vi "sub_get user input.vi"() -> (0 "Peltier Channels":i16[](array[numeric]), 1 "DAQ Sample Rate":dbl)   [LabVIEW 2021]
uses:
  globalvariables.vi
panel:
  in  "Peltier 2":i16(ring)=4 items=["N/A"=-1, "COM 1"=1, "COM 4"=4]
  in  "Peltier 1":i16(ring)=1 items=["N/A"=-1, "COM 1"=1, "COM 4"=4]
  in  "Peltier Control Mode":u16(ring) items=["Manual-Temp", "Timed-Temp", "Manual-Power", "Timed-Power", "Manual-Tamb", "Timed-Tamb"]
  in  "Valve Control Mode":u16(ring) items=["Manual-Position", "Timed-Position", "Manual-PID", "Timed-PID"]
  in  "Control Mode":i32(ring) items=["Debugger", "Manual", "Timed"]
  in  "Number of USB DAQ":i32=3
  in  "Number of Sensors":i32=32
  in  "Time Between Samples":dbl=1.0 caption="Time Between Samples (s)"
  in  "Number of Thermal Masses":i32=2
  in  "Save Directory":path=path "\\\\coeit.osu.edu\\home/b/blizard.1/Documents/Data"
  in  "Folder Name":string
  in  "Apply options":bool
  in  "Timer Length (s)":dbl
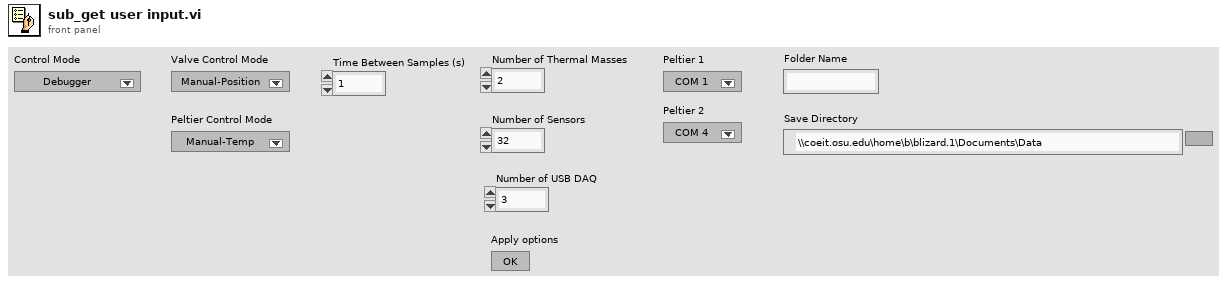
[diagram p1: front panel]
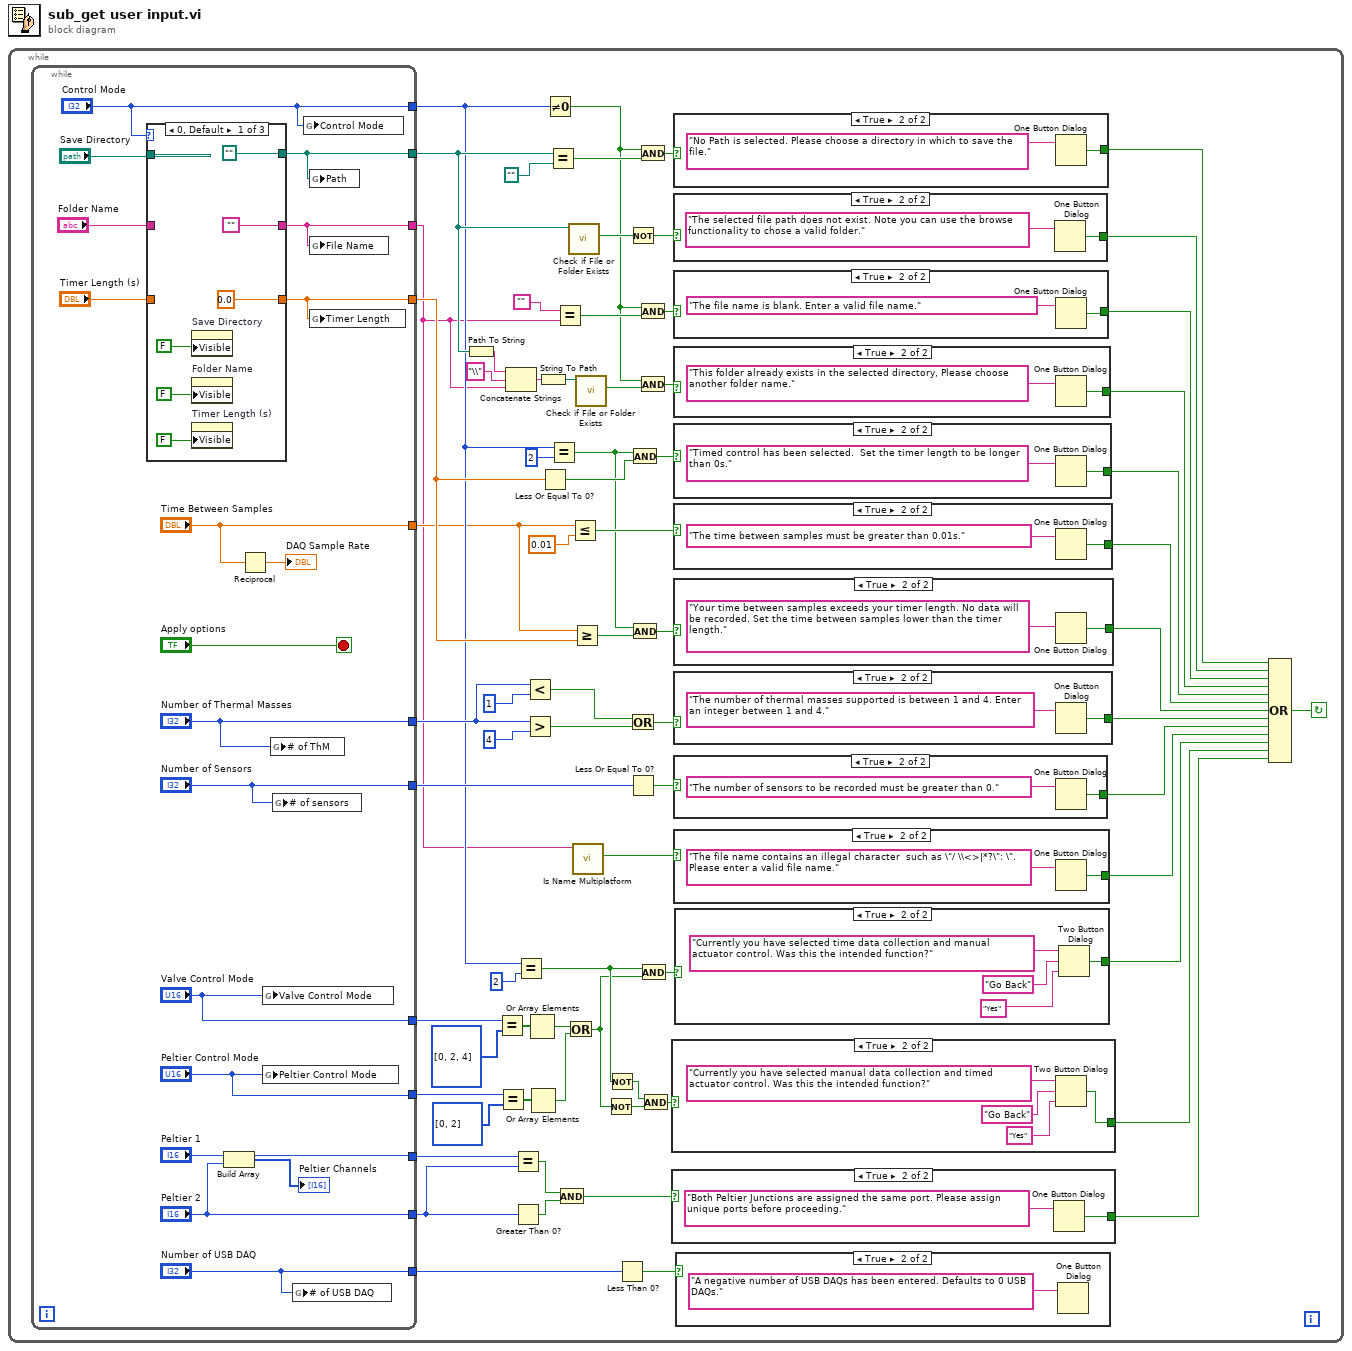
[diagram p0: block diagram]
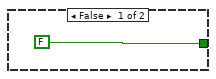
[diagram p2: hidden frame]
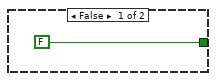
[diagram p3: hidden frame]
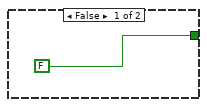
[diagram p4: hidden frame]
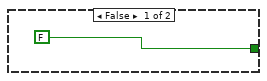
[diagram p6: hidden frame]
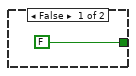
[diagram p7: hidden frame]
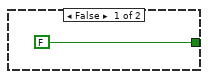
[diagram p8: hidden frame]
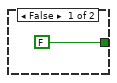
[diagram p9: hidden frame]
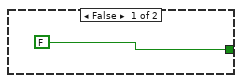
[diagram p10: hidden frame]
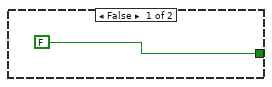
[diagram p11: hidden frame]
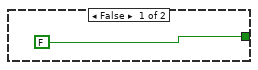
[diagram p12: hidden frame]
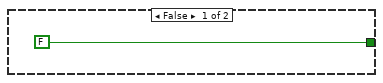
[diagram p13: hidden frame]
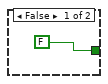
[diagram p14: hidden frame]
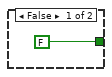
[diagram p15: hidden frame]
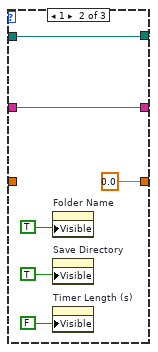
[diagram p16: hidden frame]
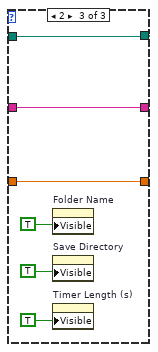
[diagram p17: hidden frame]
diagram:
  n1 = while {
    stop <- w35 continue-if-true
    n2 = while {
      tunnel: [w132] -> w28
      tunnel: [w126] -> w55
      tunnel: [w131] -> w48
      tunnel: ["Number of Thermal Masses"] -> w61
      tunnel: ["Time Between Samples"] -> w32
      tunnel: ["Number of Sensors"] -> w56
      tunnel: ["Control Mode"] -> w41
      tunnel: ["Number of USB DAQ"] -> w44
      tunnel: ["Valve Control Mode"] -> w20
      tunnel: ["Peltier Control Mode"] -> w21
      tunnel: ["Peltier 1"] -> w40
      tunnel: ["Peltier 2"] -> w39
      stop <- "Apply options" stop-if-true
      n3 = case shown="0, Default" "Control Mode" {
        tunnel: ["" w145 w151] -> w132
        tunnel: [path "" w144 w150] -> w131
        tunnel: "Folder Name" -> [_ w145 w151]
        tunnel: "Save Directory" -> [_ w144 w150]
        tunnel: [0.0 0.0 w148] -> w126
        tunnel: "Timer Length (s)" -> [_ _ w148]
        frame 0, Default {
          n4 = property on="Save Directory" class="Path"("Visible"=FALSE) -> ()  [unwired: 2 in, 2 out]
          n5 = property on="Folder Name" class="Str"("Visible"=FALSE) -> ()  [unwired: 2 in, 2 out]
          n6 = property on="Timer Length (s)" class="DigNum (strict)"("Visible"=FALSE) -> ()  [unwired: 2 in, 2 out]
        }
        frame 1 {
          n7 = property on="Folder Name" class="Str"("Visible"=TRUE) -> ()  [unwired: 2 in, 2 out]
          n8 = property on="Save Directory" class="Path"("Visible"=TRUE) -> ()  [unwired: 2 in, 2 out]
          n9 = property on="Timer Length (s)" class="DigNum (strict)"("Visible"=FALSE) -> ()  [unwired: 2 in, 2 out]
        }
        frame 2 {
          n10 = property on="Folder Name" class="Str"("Visible"=TRUE) -> ()  [unwired: 2 in, 2 out]
          n11 = property on="Save Directory" class="Path"("Visible"=TRUE) -> ()  [unwired: 2 in, 2 out]
          n12 = property on="Timer Length (s)" class="DigNum (strict)"("Visible"=TRUE) -> ()  [unwired: 2 in, 2 out]
        }
      }
      n13 = Build Array("Peltier 1", "Peltier 2") -> (→"Peltier Channels":i16[])
      n14 = Reciprocal(x="Time Between Samples") -> (1/x=→"DAQ Sample Rate":dbl)
      n15 = global write "globalvariables.vi" "Valve Control Mode"("Valve Control Mode") -> ()
      n16 = global write "globalvariables.vi" "Peltier Control Mode"("Peltier Control Mode") -> ()
      n17 = global write "globalvariables.vi" "# of ThM"("Number of Thermal Masses") -> ()
      n18 = global write "globalvariables.vi" "# of sensors"("Number of Sensors") -> ()
      n19 = global write "globalvariables.vi" "# of USB DAQ"("Number of USB DAQ") -> ()
      n20 = global write "globalvariables.vi" "Control Mode"("Control Mode") -> ()
      n21 = global write "globalvariables.vi" "Path"(w131) -> ()
      n22 = global write "globalvariables.vi" "File Name"(w132) -> ()
      n23 = global write "globalvariables.vi" "Timer Length"(w126) -> ()
    }
    n24 = Path To String(path=w48) -> (string=w68:string)
    n25 = Equal?(x=w20, y=i32[] [0, 2, 4]) -> (x = y?=w24:bool[])
    n26 = Equal?(x=w21, y=i32[] [0, 2]) -> (x = y?=w23:bool[])
    n27 = Concatenate Strings(w68, "\\", w28) -> (w67:string)
    n28 = Equal?(x=w40, y=w39) -> (x = y?=w37:bool)
    n29 = Greater Than 0?(x=w39) -> (x > 0?=w38:bool)
    n30 = Equal?(x=w41, y=2) -> (x = y?=w18:bool)
    n31 = Less?(x=w61, y=1) -> (x < y?=w60:bool)
    n32 = Greater?(x=w61, y=4) -> (0:w59:bool)
    n33 = Or Array Elements(Boolean array=w24) -> (logical OR=w17:bool)
    n34 = Or Array Elements(Boolean array=w23) -> (logical OR=w16:bool)
    n35 = String To Path(string=w67) -> (path=w33:path)
    n36 = Less Or Equal To 0?(x=w55) -> (x <= 0?=w54:bool)
    n37 = Not Equal To 0?(x=w41) -> (x != 0?=w29:bool)
    n38 = Equal?(x=w48, y=path "") -> (x = y?=w52:bool)
    n39 = Equal?(x=w41, y=2) -> (x = y?=w46:bool)
    n40 = Equal?(x="", y=w28) -> (x = y?=w47:bool)
    n41 = And(x=w37, y=w38) -> (x .and. y?=w36:bool)
    n42 = Or(x=w17, y=w16) -> (x .or. y?=w15:bool)
    n43 = call <vilib>:"Check if File or Folder Exists.vi"("path"=w48) -> ("file or folder exists?"=w65:bool)  [unwired: 8 in, 2 out]
    n44 = Less Or Equal?(x=w32, y=0.01) -> (x <= y?=w69:bool)
    n45 = Greater Or Equal?(x=w32, y=w55) -> (x >= y?=w45:bool)
    n46 = call <vilib>:"Is Name Multiplatform.vi"("filename"=w28) -> ("filename had conflict"=w27:bool)  [unwired: 6 in, 4 out]
    n47 = call <vilib>:"Check if File or Folder Exists.vi"("path"=w33) -> ("file or folder exists?"=w31:bool)  [unwired: 8 in, 2 out]
    n48 = Not(x=w15) -> (.not. x?=w26:bool)
    n49 = Not(x=w18) -> (.not. x?=w19:bool)
    n50 = Less Than 0?(x=w44) -> (x < 0?=w53:bool)
    n51 = Not(x=w65) -> (.not. x?=w64:bool)
    n52 = Or(x=w60, y=w59) -> (x .or. y?=w58:bool)
    n53 = Less Or Equal To 0?(x=w56) -> (x <= 0?=w57:bool)
    n54 = And(x=w46, y=w54) -> (x .and. y?=w72:bool)
    n55 = And(x=w46, y=w45) -> (x .and. y?=w66:bool)
    n56 = And(x=w29, y=w52) -> (x .and. y?=w51:bool)
    n57 = And(x=w29, y=w47) -> (x .and. y?=w50:bool)
    n58 = And(x=w29, y=w31) -> (x .and. y?=w30:bool)
    n59 = And(x=w18, y=w15) -> (x .and. y?=w43:bool)
    n60 = And(x=w19, y=w26) -> (x .and. y?=w42:bool)
    n61 = case shown="True" w42 {
      tunnel: [FALSE w80] -> w2
      frame False {
      }
      frame True {
        n62 = Two Button Dialog(message="Currently you have selected manual data collection and timed actuator control. Was this the intended function?", 1:"Yes", 2:"Go Back") -> (T button?=w80:bool)
      }
    }
    n63 = case shown="True" w36 {
      tunnel: [FALSE w75] -> w1
      frame False {
      }
      frame True {
        n64 = One Button Dialog(message="Both Peltier Junctions are assigned the same port. Please assign unique ports before proceeding.") -> (true=w75:bool)  [unwired: 1 in]
      }
    }
    n65 = case shown="True" w51 {
      tunnel: [FALSE w110] -> w13
      frame False {
      }
      frame True {
        n66 = One Button Dialog(message="No Path is selected. Please choose a directory in which to save the file.") -> (true=w110:bool)  [unwired: 1 in]
      }
    }
    n67 = case shown="True" w64 {
      tunnel: [FALSE w92] -> w12
      frame False {
      }
      frame True {
        n68 = One Button Dialog(message="The selected file path does not exist. Note you can use the browse functionality to chose a valid folder.") -> (true=w92:bool)  [unwired: 1 in]
      }
    }
    n69 = case shown="True" w50 {
      tunnel: [FALSE w117] -> w11
      frame False {
      }
      frame True {
        n70 = One Button Dialog(message="The file name is blank. Enter a valid file name.") -> (true=w117:bool)  [unwired: 1 in]
      }
    }
    n71 = case shown="True" w30 {
      tunnel: [FALSE w101] -> w10
      frame False {
      }
      frame True {
        n72 = One Button Dialog(message="This folder already exists in the selected directory, Please choose another folder name.") -> (true=w101:bool)  [unwired: 1 in]
      }
    }
    n73 = case shown="True" w72 {
      tunnel: [FALSE w114] -> w9
      frame False {
      }
      frame True {
        n74 = One Button Dialog(message="Timed control has been selected.  Set the timer length to be longer than 0s.") -> (true=w114:bool)  [unwired: 1 in]
      }
    }
    n75 = case shown="True" w69 {
      tunnel: [FALSE w107] -> w8
      frame False {
      }
      frame True {
        n76 = One Button Dialog(message="The time between samples must be greater than 0.01s.") -> (true=w107:bool)  [unwired: 1 in]
      }
    }
    n77 = case shown="True" w66 {
      tunnel: [FALSE w98] -> w7
      frame False {
      }
      frame True {
        n78 = One Button Dialog(message="Your time between samples exceeds your timer length. No data will be recorded. Set the time between samples lower than the timer length.") -> (true=w98:bool)  [unwired: 1 in]
      }
    }
    n79 = case shown="True" w58 {
      tunnel: [FALSE w104] -> w6
      frame False {
      }
      frame True {
        n80 = One Button Dialog(message="The number of thermal masses supported is between 1 and 4. Enter an integer between 1 and 4.") -> (true=w104:bool)  [unwired: 1 in]
      }
    }
    n81 = case shown="True" w57 {
      tunnel: [FALSE w89] -> w5
      frame False {
      }
      frame True {
        n82 = One Button Dialog(message="The number of sensors to be recorded must be greater than 0.") -> (true=w89:bool)  [unwired: 1 in]
      }
    }
    n83 = case shown="True" w27 {
      tunnel: [FALSE w95] -> w4
      frame False {
      }
      frame True {
        n84 = One Button Dialog(message="The file name contains an illegal character  such as \"/ \\<>|*?\": \". Please enter a valid file name.") -> (true=w95:bool)  [unwired: 1 in]
      }
    }
    n85 = case shown="True" w43 {
      tunnel: [FALSE w85] -> w3
      frame False {
      }
      frame True {
        n86 = Two Button Dialog(message="Currently you have selected time data collection and manual actuator control. Was this the intended function?", 1:"Yes", 2:"Go Back") -> (T button?=w85:bool)
      }
    }
    n87 = case shown="True" w53 {
      frame False {
      }
      frame True {
        n88 = One Button Dialog(message="A negative number of USB DAQs has been entered. Defaults to 0 USB DAQs.") -> ()  [unwired: 1 in, 1 out]
      }
    }
    n89 = Compound Arithmetic op=OR(w13, w12, w11, w10, w9, w8, w7, w6, w5, w4, w3, w2, w1) -> (w35:bool)
  }
